vi "VCS Read Data Buffer.vi"(6 "error in (no error)":errorcluster, 7 "BufferSizeToRead":u32, 9 "axis in":cluster{"keyHandle":u32, "nodeId":u16}={"keyHandle"=0, "nodeId"=1}) -> (0 "error out":errorcluster, 1 "data buffer":T1, 3 "axis out":cluster{"keyHandle":u32, "nodeId":u16}={"keyHandle"=0, "nodeId"=1})   [LabVIEW 2017, in "maxonEPOS.lvlib"]
doc: "<B>VCS_ReadDataBuffer</B> returns the buffer data points."
uses:
  Examples/maxonEPOS.lvlib
  SSI_Tool/InstrumentsInterfaces/Motordriver/maxon EPOS/Resources/EposCmd.dll
  SSI_Tool/InstrumentsInterfaces/Motordriver/maxon EPOS/Resources/EposCmd64.dll
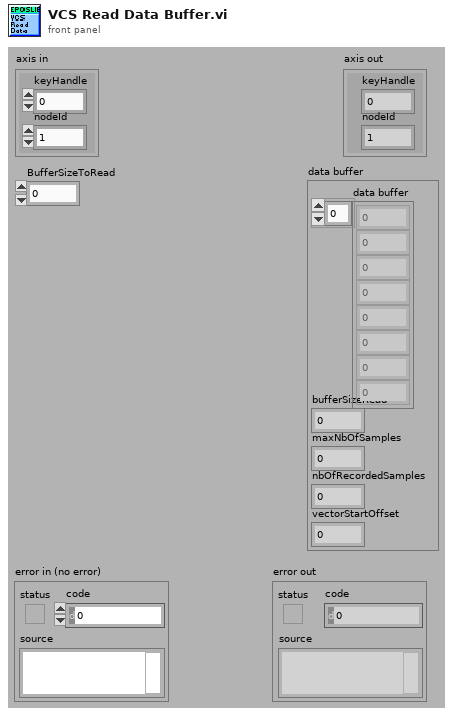
[diagram p1: front panel]
types:
  T1 = cluster{"bufferSizeRead":u32, "vectorStartOffset":u16, "maxNbOfSamples":u16, "nbOfRecordedSamples":u16, "data buffer":u8[]}
  T2 = cluster{"pBufferSizeRead":u32, "pVectorStartOffset":u16, "pMaxNbOfSamples":u16, "pNbOfRecordedSamples":u16, "pDataBuffer":u8[]}
  T3 = cluster{"bufferSizeRead":u32, "vectorStartOffset":u16, "maxNbOfSamples":u16, "nbOfRecordedSamples":u16, u8[]}
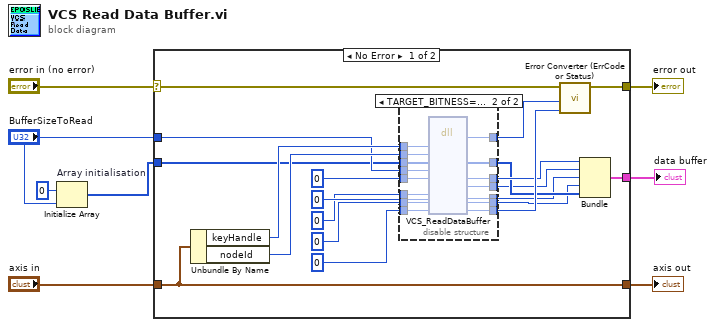
[diagram p0: block diagram]
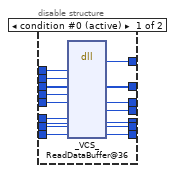
[diagram p2: hidden frame]
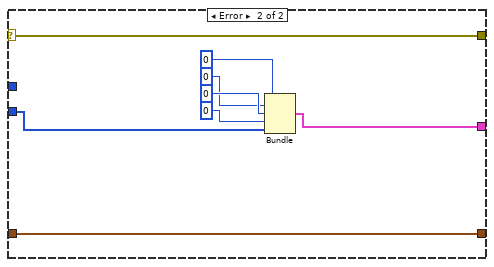
[diagram p3: hidden frame]
diagram:
  n1 = Initialize Array "Array initialisation"(u8 0, "BufferSizeToRead") -> (w2:u8[])
  n2 = case shown="No Error" "error in (no error)" {
    selector: "error in (no error)" -> [w26 w67]
    tunnel: "axis in" -> [w28 w68]
    tunnel: [w28 w68] -> w7
    tunnel: [w27 w67] -> w6
    tunnel: "BufferSizeToRead" -> [w20 _]
    tunnel: w2 -> [w19 w66]
    tunnel: [w9 w61] -> w1
    frame No Error {
      n3 = Unbundle By Name(w28) -> ("keyHandle"=w21:u32, "nodeId"=w22:u16)
      n4 = disable-structure shown="TARGET_BITNESS==64" {
        disable-tunnel: u32 0 ("pErrorCode") -> [w44 w60]
        disable-tunnel: [w43 w59] -> w24
        disable-tunnel: [w42 w58] -> w23
        disable-tunnel: w22 -> [w41 w57]
        disable-tunnel: w21 -> [w40 w56]
        disable-tunnel: w20 -> [w39 w55]
        disable-tunnel: w19 -> [w38 w54]
        disable-tunnel: u32 0 ("pBufferSizeRead") -> [w37 w53]
        disable-tunnel: u16 0 ("pVectorStartOffset") -> [w36 w52]
        disable-tunnel: u16 0 ("pMaxNbOfSamples") -> [w35 w51]
        disable-tunnel: u16 0 ("pNbOfRecordedSamples") -> [w34 w50]
        disable-tunnel: [w33 w49] -> w14
        disable-tunnel: [w32 w48] -> w13
        disable-tunnel: [w31 w47] -> w12
        disable-tunnel: [w30 w46] -> w11
        disable-tunnel: [w29 w45] -> w10
        frame condition #0 (active) {
          n5 = dll-call lib="C:/workspace/project/scancon/sw/SSI_Tool/InstrumentsInterfaces/Motordriver/maxon EPOS/Resources/EposCmd.*" fn="_VCS_ReadDataBuffer@36" ("VCS_ReadDataBuffer")("KeyHandle"=w40, "NodeId"=w41, "pDataBuffer"=w38, "BufferSizeToRead"=w39, "pBufferSizeRead"=w37, "pVectorStartOffset"=w36, "pMaxNbOfSamples"=w35, "pNbOfRecordedSamples"=w34, "pErrorCode"=w44) -> ("Rückgabetyp"=w42:i32, "pDataBuffer"=w32:u8[], "pBufferSizeRead"=w33:u32, "pVectorStartOffset"=w31:u16, "pMaxNbOfSamples"=w30:u16, "pNbOfRecordedSamples"=w29:u16, "pErrorCode"=w43:u32)  [unwired: 6 in, 2 out]
        }
        frame condition #1 {
          n6 = dll-call lib="C:/setup/Resources/EposCmd64.*" fn="VCS_ReadDataBuffer"("KeyHandle"=w56, "NodeId"=w57, "pDataBuffer"=w54, "BufferSizeToRead"=w55, "pBufferSizeRead"=w53, "pVectorStartOffset"=w52, "pMaxNbOfSamples"=w51, "pNbOfRecordedSamples"=w50, "pErrorCode"=w60) -> ("Rückgabetyp"=w58:i32, "pDataBuffer"=w48:u8[], "pBufferSizeRead"=w49:u32, "pVectorStartOffset"=w47:u16, "pMaxNbOfSamples"=w46:u16, "pNbOfRecordedSamples"=w45:u16, "pErrorCode"=w59:u32)  [unwired: 6 in, 2 out]
        }
      }
      n7 = call "Error Converter (ErrCode or Status).vi"("error code"=w24, "return type"=w23, "error in (no error)"=w26) -> ("error out"=w27:errorcluster)  [unwired: 7 in]
      n8 = Bundle("pBufferSizeRead"=w14, "pVectorStartOffset"=w12, "pMaxNbOfSamples"=w11, "pNbOfRecordedSamples"=w10, "pDataBuffer"=w13) -> (w9:T2)  [unwired: 1 in]
    }
    frame Error {
      n9 = Bundle("bufferSizeRead"=u32 0, "vectorStartOffset"=u16 0, "maxNbOfSamples"=u16 0, "nbOfRecordedSamples"=u16 0, w66) -> (w61:T3)  [unwired: 1 in]
    }
  }
  "error out" <- w6
  "axis out" <- w7
  "data buffer" <- w1
